vi "Q_Get Total Distance in KM.vi"(8 "error in (no error)":errorcluster, 11 "Data Manager in":refnum<class "Data Manager.lvclass">) -> (0 "error out":errorcluster, 1 "Group B":dbl, 2 "Group A":dbl, 3 "Data Manager out":refnum<class "Data Manager.lvclass">, 5 "Total":dbl)   [LabVIEW 2020, in "Data Manager.lvclass"]
uses:
  Data Manager.lvclass
  Data Manager.lvclass/Data Manager.ctl
  <vilib>/drjdpowell/SQLite Library/SQL Connection/Execute SQL (DBL results).vi
  <vilib>/drjdpowell/SQLite Library/SQLite.lvlib
  <vilib>/drjdpowell/SQLite Library/SQL Connection/Connection.lvclass
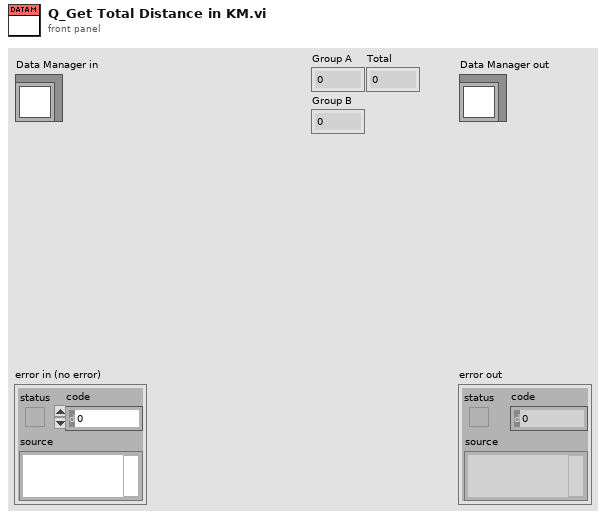
[diagram p1: front panel]
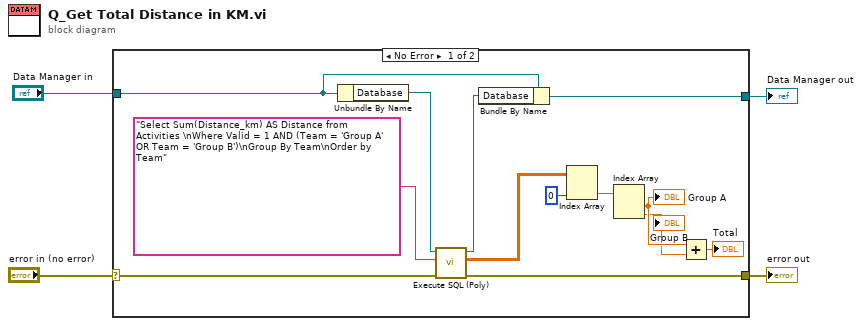
[diagram p0: block diagram]
diagram:
  n1 = case shown="No Error" "error in (no error)" {
    selector: "error in (no error)" -> [w13 w19]
    tunnel: [w12 w19] -> w3
    tunnel: [w15 w18] -> w1
    tunnel: "Data Manager in" -> [w16 w18]
    frame No Error {
      n2 = Unbundle By Name(w16) -> ("Database"=w17:refnum<class "Connection.lvclass">)
      n3 = call-poly <vilib>:"Execute SQL (Poly).vi"("error in (no error)"=w13, "SQL"="Select Sum(Distance_km) AS Distance from Activities \nWhere Valid = 1 AND (Team = 'Group A' OR Team = 'Group B')\nGroup By Team\nOrder by Team", "SQLite Connection in"=w17) -> ("error out"=w12:errorcluster, "Result Set"=w10:dbl[][], "SQLite Connection"=w14:refnum<class "Connection.lvclass">)  [unwired: 5 in, 1 out]
      n4 = Bundle By Name(cluster=w16, "Database"=w14) -> (w15:refnum<class "Data Manager.lvclass">)
      n5 = Index Array(array=w10, index (col)=0 ("disabled index (col)")) -> (element=w8:dbl[])  [unwired: 1 in]
      n6 = Index Array(array=w8) -> (element #1=w7:dbl, element #2=w6:dbl)  [unwired: 2 in]
      "Group A" <- w7
      "Group B" <- w6
      n7 = Add(x=w7, y=w6) -> (x+y=→"Total":dbl)
    }
    frame Error {
    }
  }
  "error out" <- w3
  "Data Manager out" <- w1
